vi "String Replace LabVIEW Data Types With C types.vi"(1 "C code":string) -> (0 "C code, replaced datatypes":string)   [LabVIEW 2014]
doc: "Concatenates String Array Into one String. If optional delimiter provided, it's inserted between each String Array item."
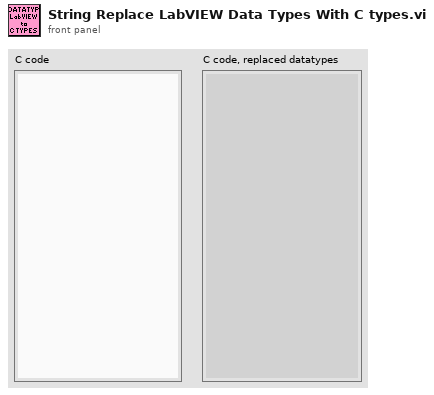
[diagram p1: front panel]
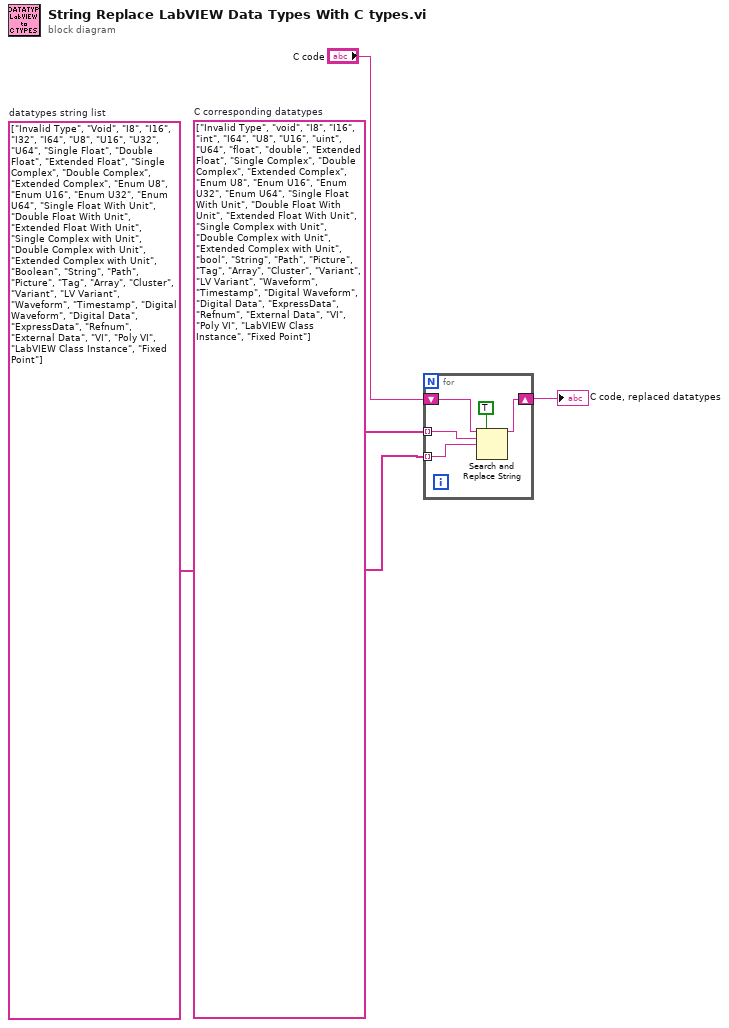
[diagram p0: block diagram]
diagram:
  w3 = string[] ["Invalid Type", "void", "I8", "I16", "int", "I64", "U8", "U16", "uint", "U64", "float", "double", "Extended Float", "Single Complex", "Double Complex", "Extended Complex", "Enum U8", "Enum U16", "Enum U32", "Enum U64", "Single Float With Unit", "Double Float With Unit", "Extended Float With Unit", "Single Complex with Unit", "Double Complex with Unit", "Extended Complex with Unit", "bool", "String", "Path", "Picture", "Tag", "Array", "Cluster", "Variant", "LV Variant", "Waveform", "Timestamp", "Digital Waveform", "Digital Data", "ExpressData", "Refnum", "External Data", "VI", "Poly VI", "LabVIEW Class Instance", "Fixed Point"]  # C corresponding datatypes
  w4 = string[] ["Invalid Type", "Void", "I8", "I16", "I32", "I64", "U8", "U16", "U32", "U64", "Single Float", "Double Float", "Extended Float", "Single Complex", "Double Complex", "Extended Complex", "Enum U8", "Enum U16", "Enum U32", "Enum U64", "Single Float With Unit", "Double Float With Unit", "Extended Float With Unit", "Single Complex with Unit", "Double Complex with Unit", "Extended Complex with Unit", "Boolean", "String", "Path", "Picture", "Tag", "Array", "Cluster", "Variant", "LV Variant", "Waveform", "Timestamp", "Digital Waveform", "Digital Data", "ExpressData", "Refnum", "External Data", "VI", "Poly VI", "LabVIEW Class Instance", "Fixed Point"]  # datatypes string list
  n1 = for {
    tunnel: w4 -> [w8] mode=indexing
    tunnel: w3 -> [w7] mode=indexing
    shift-right: [w5] -> w1
    shift-left: "C code" -> [w9]
    n2 = Search and Replace String(replace all?=TRUE ("replace all? (F)"), input string=w9, search string=w8, replace string=w7) -> (result string=w5:string)  [unwired: 4 in, 3 out]
  }
  "C code, replaced datatypes" <- w1
